vi "ROM chip.vi"(1 "Clock":bool, 2 "Address":bool[](array[boolean])=[FALSE, FALSE, FALSE, FALSE, FALSE, FALSE, FALSE, FALSE, FALSE, FALSE, FALSE, FALSE, FALSE, FALSE, FALSE, FALSE]) -> (0 "Reg Out":bool[](array[boolean]))   [LabVIEW 2012]
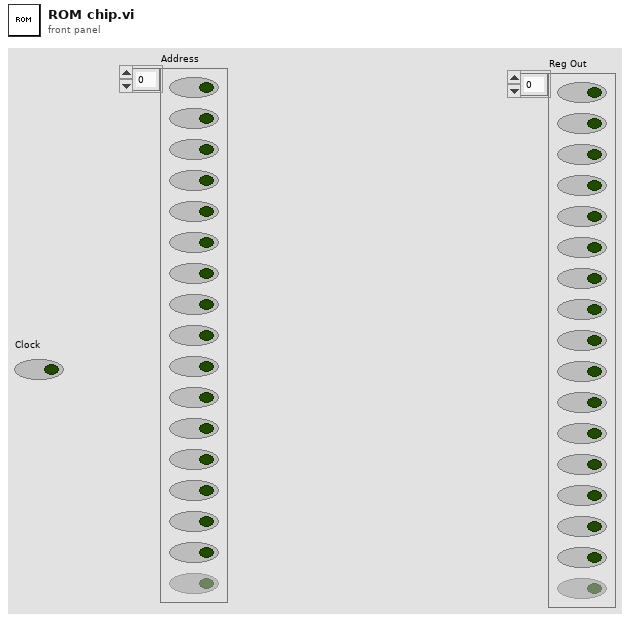
[diagram p1: front panel]
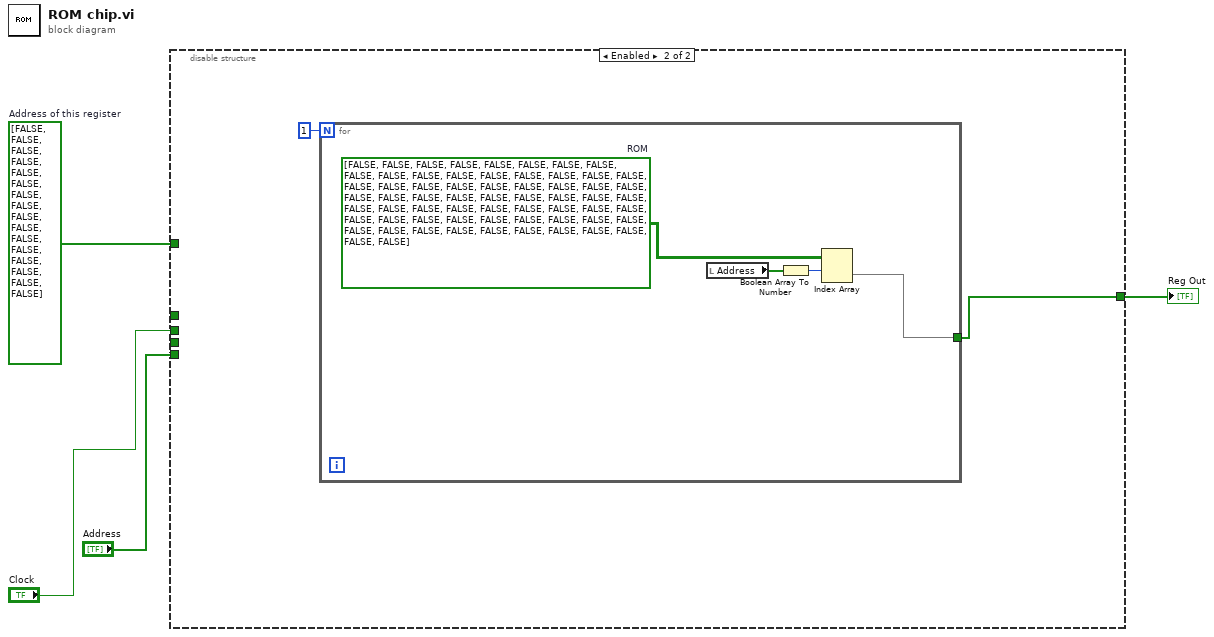
[diagram p0: block diagram]
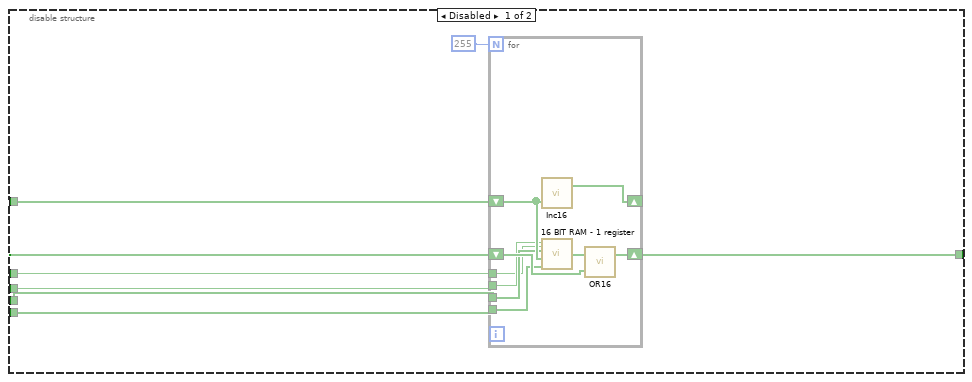
[diagram p2: hidden frame]
diagram:
  w4 = bool[] [FALSE, FALSE, FALSE, FALSE, FALSE, FALSE, FALSE, FALSE, FALSE, FALSE, FALSE, FALSE, FALSE, FALSE, FALSE, FALSE]  # Address of this register
  n1 = disable-structure shown="Enabled" {
    disable-tunnel: w4 -> [w11 _]
    disable-tunnel: [w10 w21] -> w3
    disable-tunnel: "Clock" -> [w8 _]
    disable-tunnel: "Address" -> [w7 _]
    disable-tunnel: _ -> [w6 _]
    disable-tunnel: _ -> [w5 _]
    frame Disabled {
      n2 = for {
        N: u16 255 -> [_]
        shift-right: [w19] -> _
        shift-left: w11 -> [w20]
        shift-right: [w16] -> w10
        shift-left: w11 -> [w18]
        tunnel: w8 -> [w15]
        tunnel: w7 -> [w14]
        tunnel: w5 -> [w12]
        tunnel: w6 -> [w13]
        n3 = call "Inc16.vi"("A"=w20) -> ("S"=w19:bool[])  [unwired: 1 in, 1 out]
        n4 = call "16 BIT RAM - 1 register.vi"("Hold"=w12, "Address"=w14, "Address of this register"=w20, "Data In"=w13, "Clock"=w15) -> ("z"=w17:bool[])  [unwired: 1 in]
        n5 = call "OR16.vi"("B"=w18, "A"=w17) -> ("z"=w16:bool[])  [unwired: 1 out]
      }
    }
    frame Enabled {
      n6 = for {
        N: 1 -> [_]
        tunnel: [w23] -> w21
        w24 = bool[][] [[FALSE, FALSE, FALSE, FALSE, FALSE, FALSE, FALSE, FALSE, FALSE, FALSE, FALSE, FALSE, FALSE, FALSE, FALSE, FALSE], [FALSE, FALSE, FALSE, FALSE, FALSE, FALSE, FALSE, FALSE, FALSE, FALSE, FALSE, FALSE, FALSE, FALSE, FALSE, FALSE], [FALSE, FALSE, FALSE, FALSE, FALSE, FALSE, FALSE, FALSE, FALSE, FALSE, FALSE, FALSE, FALSE, FALSE, FALSE, FALSE], [FALSE, FALSE, FALSE, FALSE, FALSE, FALSE, FALSE, FALSE, FALSE, FALSE, FALSE, FALSE, FALSE, FALSE, FALSE, FALSE]]  # ROM
        n7 = local read "Address"() -> (w26:bool[])
        n8 = Boolean Array To Number(Boolean array=w26) -> (number=w25:u32)
        n9 = Index Array(array=w24, index (row)=w25) -> (element=w23:bool[])  [unwired: 1 in]
      }
    }
  }
  "Reg Out" <- w3
